vi "Handle Transition to State Change.vi"(0 "action queue in":refnum<queue>, 1 "TLB' Template in":refnum<class "Synchronize AWS S3 Content TLB`.lvclass">, 5 "Destination State":T1, 11 "error in (no error)":errorcluster) -> (3 "TLB' Template out":refnum<class "Synchronize AWS S3 Content TLB`.lvclass">, 4 "action queue in":refnum<queue>, 15 "error out":errorcluster)   [LabVIEW 2026, in "Synchronize AWS S3 Content.lvlib" / "Synchronize AWS S3 Content TLB`.lvclass"]
uses:
  Synchronize AWS S3 Content TLB`.lvclass
  Actions/System Action Element.ctl
  State Machine/State.ctl
  Synchronize AWS S3 Content TLB`.lvclass/Synchronize AWS S3 Content TLB`.ctl
  Actions/Actions.lvlib
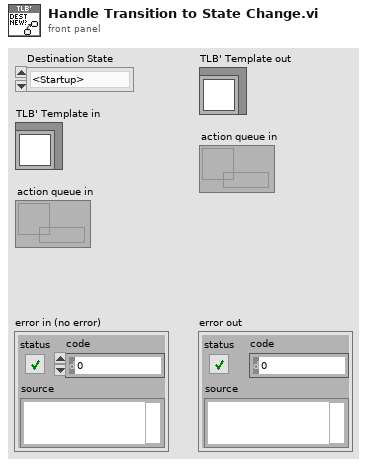
[diagram p1: front panel]
types:
  T1 = typedef "Synchronize AWS S3 Content.lvlib/Synchronize AWS S3 Content TLB`.lvclass/State.ctl" = enum16{"<Startup>", "Idle", "Initiating Configuration", "Validating Commands", "Executing Synchronization", "Validation", "<Shutdown>", "<Error>"}
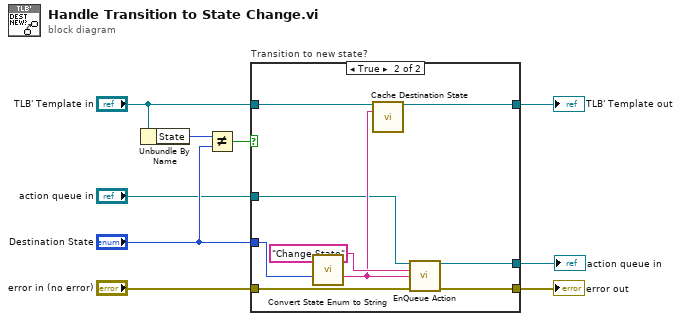
[diagram p0: block diagram]
diagram:
  n1 = Unbundle By Name("TLB' Template in") -> ("State"=w1:T1)
  n2 = Not Equal?(x=w1, y="Destination State") -> (x != y?=w8:bool)
  n3 = case "Transition to new state?" shown="True" w8 {
    tunnel: "action queue in" -> [w11 w13]
    tunnel: "error in (no error)" -> [w12 w20]
    tunnel: [w12 w19] -> w6
    tunnel: "Destination State" -> [_ w18]
    tunnel: [w11 w21] -> w7
    tunnel: "TLB' Template in" -> [w10 w15]
    tunnel: [w10 w14] -> w9
    frame False {
    }
    frame True {
      n4 = call "Convert State Enum to String.vi"("state in"=w18) -> ("state out"=w16:string)  [unwired: 13 in, 1 out]
      n5 = call "Cache Destination State.vi"("TLB' Template in"=w15, "state in"=w16) -> ("TLB' Template out"=w14:refnum<class "Synchronize AWS S3 Content TLB`.lvclass">)  [unwired: 13 in]
      n6 = call "EnQueue Action.vi"("action queue in"=w13, "action"="Change State" ("Message Name"), "data in"=w16, "error in"=w20) -> ("action queue out"=w21:refnum<queue>, "error out"=w19:errorcluster)  [unwired: 10 in]
    }
  }
  "TLB' Template out" <- w9
  "action queue in" <- w7
  "error out" <- w6
